vi "Калькулятор.vi"() -> ()   [LabVIEW 2012]
uses:
  Control 1.ctl
panel:
  in  "Backsppace":bool
  in  "CE":bool
  in  "+/-":bool
  in  ",":bool
  in  "1/x":bool
  in  "кв":bool
  in  "к":bool
  in  "MC":bool
  out "Boolean":bool
  in  "MR":bool
  in  "-":bool
  in  "6":bool
  in  "5":bool
  in  "4":bool
  in  "MS":bool
  in  "С":bool
  in  "/":bool
  in  "*":bool
  in  "0":bool
  in  "9":bool
  in  "8":bool
  in  "7":bool
  in  "3":bool
  in  "stop":bool
  in  "=":bool
  in  "2":bool
  in  "+":bool
  out "екран":string
  in  "1":bool
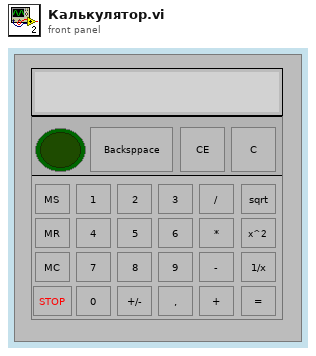
[diagram p1: front panel]
types:
  T1 = typedef "Control 1.ctl" = enum16{"Backspace", "се", "+/-", "т", "1/x", "кв", "к", "mc", "mr", "очистити екран", "ms", "поділити", "помножити", "відняти", "0", "9", "8", "7", "6", "5", "4", "3", "дорівнює", "додати", "2", "1", "евент", "стоп"}
  T2 = cluster{"екран":string, "чистий екран":string, "буфер":string, "Enum":T1, "ms":string, "mr ":string}
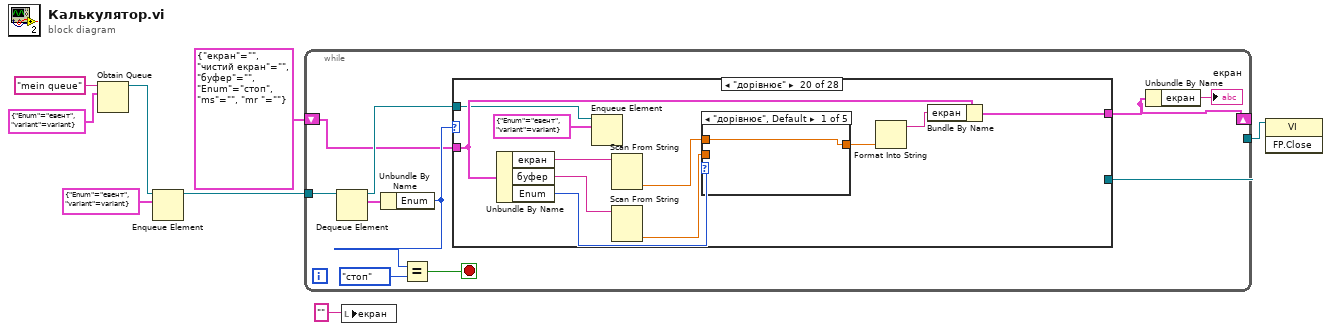
[diagram p0: block diagram]
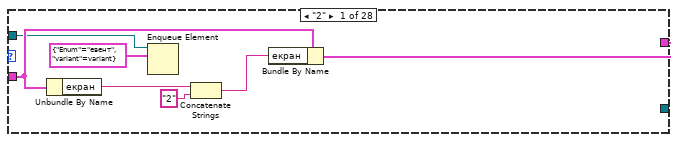
[diagram p2: hidden frame]
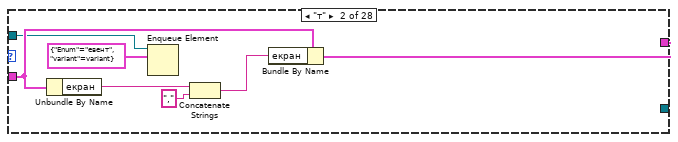
[diagram p3: hidden frame]
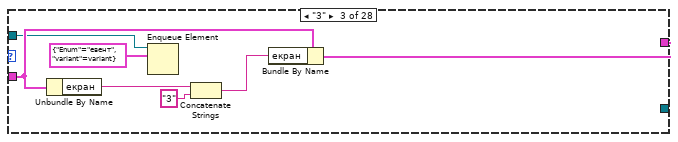
[diagram p4: hidden frame]
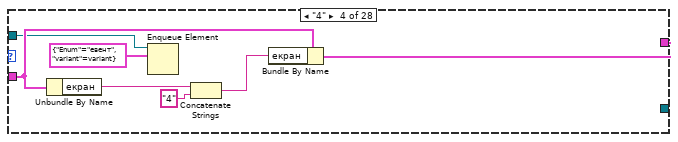
[diagram p5: hidden frame]
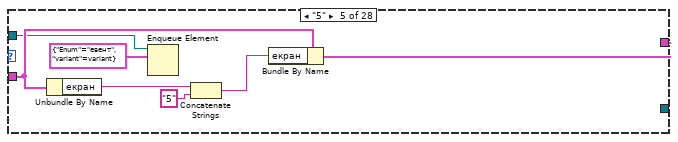
[diagram p6: hidden frame]
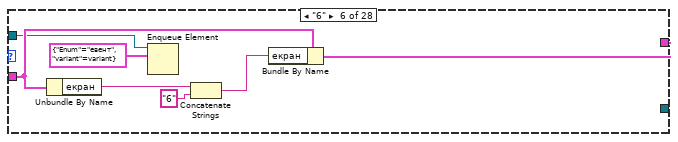
[diagram p7: hidden frame]
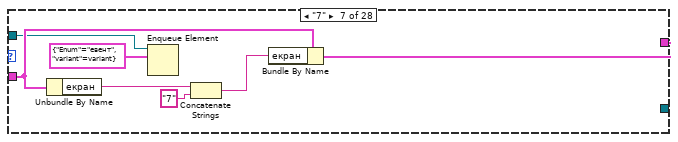
[diagram p8: hidden frame]
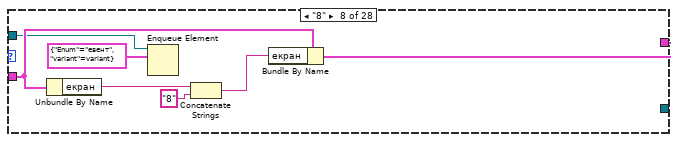
[diagram p9: hidden frame]
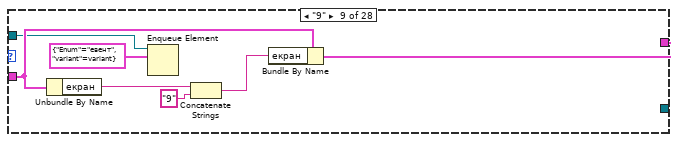
[diagram p10: hidden frame]
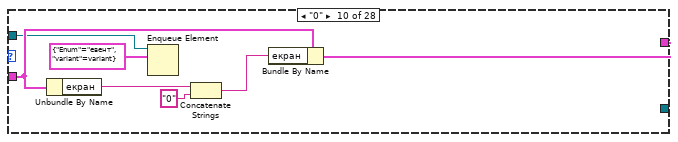
[diagram p11: hidden frame]
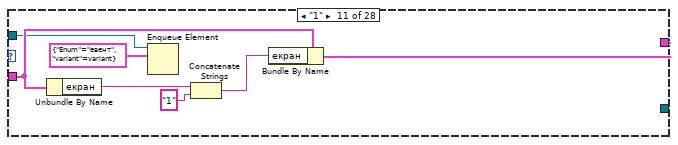
[diagram p12: hidden frame]
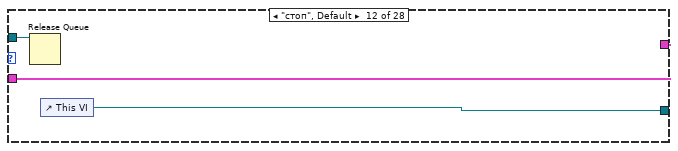
[diagram p13: hidden frame]
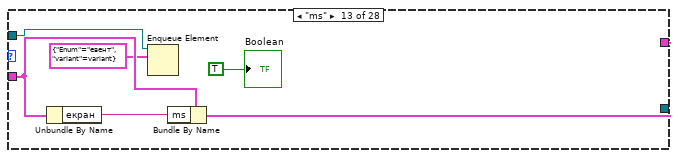
[diagram p14: hidden frame]
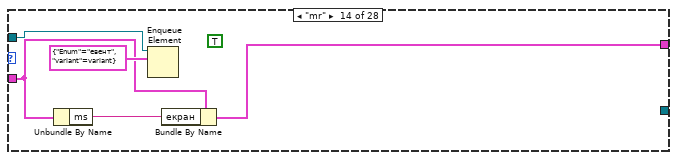
[diagram p15: hidden frame]
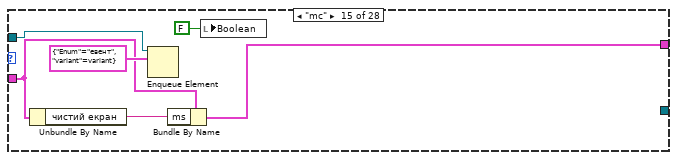
[diagram p16: hidden frame]
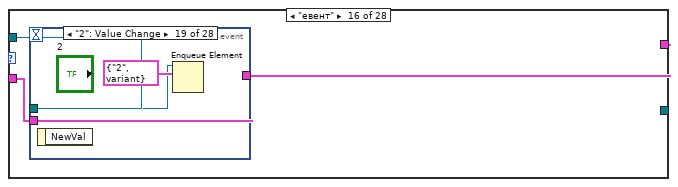
[diagram p17: hidden frame]
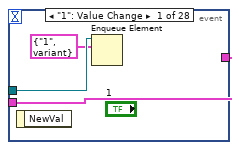
[diagram p18: hidden frame]
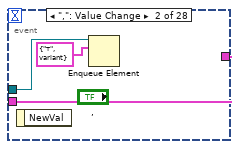
[diagram p19: hidden frame]
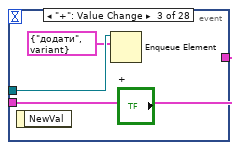
[diagram p20: hidden frame]
diagram:
  n1 = Obtain Queue(name (unnamed)="mein queue", element data type=cluster{"Enum":T1, "variant":variant} {"Enum"=enum."евент", "variant"=variant}) -> (queue out=w7:refnum<queue>)  [unwired: 3 in, 2 out]
  n2 = Enqueue Element(queue=w7, element=cluster{"Enum":T1, "variant":variant} {"Enum"=enum."евент", "variant"=variant}) -> (queue out=w4:refnum<queue>)  [unwired: 2 in, 2 out]
  n3 = while {
    tunnel: w4 -> [w16]
    shift-right: [w11] -> _
    shift-left: T2 {"екран"="", "чистий екран"="", "буфер"="", "Enum"=enum."стоп", "ms"="", "mr "=""} -> [w12]
    tunnel: [w9] -> w2
    stop <- w17 stop-if-true
    n4 = Dequeue Element(queue=w16) -> (queue out=w13:refnum<queue>, element=w15:cluster{"Enum":T1, "variant":variant})  [unwired: 2 in, 2 out]
    n5 = Unbundle By Name(w15) -> ("Enum"=w14:T1)
    n6 = Equal?(x=w14, y=Control_1."стоп" ("Enum")) -> (x = y?=w17:bool)
    n7 = case shown="\"дорівнює\"" w14 {
      tunnel: w13 -> [w20 w27 w34 w41 w48 w55 w62 w69 w76 w83 w90 w97 w100 w109 w115 w118 w237 w238 w250 w253 w282 w284 w297 w309 w317 w324 w331 w338]
      tunnel: w12 -> [w23 w30 w37 w44 w51 w58 w65 w72 w79 w86 w93 w98 w104 w106 w112 w116 w235 w242 w246 w257 w281 w286 w296 w308 w316 w323 w330 w337]
      tunnel: [w22 w29 w36 w43 w50 w57 w64 w71 w78 w85 w91 w98 w103 w105 w111 w117 w234 w240 w244 w256 w276 w285 w294 w306 w314 w318 w325 w332] -> w11
      tunnel: [_ _ _ _ _ _ _ _ _ _ _ w96 _ _ _ _ _ _ _ _ _ _ _ _ _ _ _ _] -> w9
      frame "2" {
        n8 = Unbundle By Name(w23) -> ("екран"=w25:string)
        n9 = Enqueue Element(queue=w20, element=cluster{"Enum":T1, "variant":variant} {"Enum"=enum."евент", "variant"=variant}) -> ()  [unwired: 2 in, 3 out]
        n10 = Concatenate Strings(w25, "2" ("string")) -> (w21:string)
        n11 = Bundle By Name(cluster=w23, "екран"=w21) -> (w22:T2)
      }
      frame "т" {
        n12 = Unbundle By Name(w30) -> ("екран"=w32:string)
        n13 = Enqueue Element(queue=w27, element=cluster{"Enum":T1, "variant":variant} {"Enum"=enum."евент", "variant"=variant}) -> ()  [unwired: 2 in, 3 out]
        n14 = Concatenate Strings(w32, "," ("string")) -> (w28:string)
        n15 = Bundle By Name(cluster=w30, "екран"=w28) -> (w29:T2)
      }
      frame "3" {
        n16 = Unbundle By Name(w37) -> ("екран"=w39:string)
        n17 = Enqueue Element(queue=w34, element=cluster{"Enum":T1, "variant":variant} {"Enum"=enum."евент", "variant"=variant}) -> ()  [unwired: 2 in, 3 out]
        n18 = Concatenate Strings(w39, "3" ("string")) -> (w35:string)
        n19 = Bundle By Name(cluster=w37, "екран"=w35) -> (w36:T2)
      }
      frame "4" {
        n20 = Unbundle By Name(w44) -> ("екран"=w46:string)
        n21 = Enqueue Element(queue=w41, element=cluster{"Enum":T1, "variant":variant} {"Enum"=enum."евент", "variant"=variant}) -> ()  [unwired: 2 in, 3 out]
        n22 = Concatenate Strings(w46, "4" ("string")) -> (w42:string)
        n23 = Bundle By Name(cluster=w44, "екран"=w42) -> (w43:T2)
      }
      frame "5" {
        n24 = Unbundle By Name(w51) -> ("екран"=w53:string)
        n25 = Enqueue Element(queue=w48, element=cluster{"Enum":T1, "variant":variant} {"Enum"=enum."евент", "variant"=variant}) -> ()  [unwired: 2 in, 3 out]
        n26 = Concatenate Strings(w53, "5" ("string")) -> (w49:string)
        n27 = Bundle By Name(cluster=w51, "екран"=w49) -> (w50:T2)
      }
      frame "6" {
        n28 = Unbundle By Name(w58) -> ("екран"=w60:string)
        n29 = Enqueue Element(queue=w55, element=cluster{"Enum":T1, "variant":variant} {"Enum"=enum."евент", "variant"=variant}) -> ()  [unwired: 2 in, 3 out]
        n30 = Concatenate Strings(w60, "6" ("string")) -> (w56:string)
        n31 = Bundle By Name(cluster=w58, "екран"=w56) -> (w57:T2)
      }
      frame "7" {
        n32 = Unbundle By Name(w65) -> ("екран"=w67:string)
        n33 = Enqueue Element(queue=w62, element=cluster{"Enum":T1, "variant":variant} {"Enum"=enum."евент", "variant"=variant}) -> ()  [unwired: 2 in, 3 out]
        n34 = Concatenate Strings(w67, "7" ("string")) -> (w63:string)
        n35 = Bundle By Name(cluster=w65, "екран"=w63) -> (w64:T2)
      }
      frame "8" {
        n36 = Unbundle By Name(w72) -> ("екран"=w74:string)
        n37 = Enqueue Element(queue=w69, element=cluster{"Enum":T1, "variant":variant} {"Enum"=enum."евент", "variant"=variant}) -> ()  [unwired: 2 in, 3 out]
        n38 = Concatenate Strings(w74, "8" ("string")) -> (w70:string)
        n39 = Bundle By Name(cluster=w72, "екран"=w70) -> (w71:T2)
      }
      frame "9" {
        n40 = Unbundle By Name(w79) -> ("екран"=w81:string)
        n41 = Enqueue Element(queue=w76, element=cluster{"Enum":T1, "variant":variant} {"Enum"=enum."евент", "variant"=variant}) -> ()  [unwired: 2 in, 3 out]
        n42 = Concatenate Strings(w81, "9" ("string")) -> (w77:string)
        n43 = Bundle By Name(cluster=w79, "екран"=w77) -> (w78:T2)
      }
      frame "0" {
        n44 = Unbundle By Name(w86) -> ("екран"=w88:string)
        n45 = Enqueue Element(queue=w83, element=cluster{"Enum":T1, "variant":variant} {"Enum"=enum."евент", "variant"=variant}) -> ()  [unwired: 2 in, 3 out]
        n46 = Concatenate Strings(w88, "0" ("string")) -> (w84:string)
        n47 = Bundle By Name(cluster=w86, "екран"=w84) -> (w85:T2)
      }
      frame "1" {
        n48 = Unbundle By Name(w93) -> ("екран"=w95:string)
        n49 = Enqueue Element(queue=w90, element=cluster{"Enum":T1, "variant":variant} {"Enum"=enum."евент", "variant"=variant}) -> ()  [unwired: 2 in, 3 out]
        n50 = Concatenate Strings(w95, "1" ("string")) -> (w92:string)
        n51 = Bundle By Name(cluster=w93, "екран"=w92) -> (w91:T2)
      }
      frame "стоп", Default {
        n52 = Release Queue(queue=w97) -> ()  [unwired: 2 in, 3 out]
        n53 = control-ref of="This VI"() -> (w96:refnum<vi>)
      }
      frame "ms" {
        n54 = Unbundle By Name(w104) -> ("екран"=w101:string)
        n55 = Enqueue Element(queue=w100, element=cluster{"Enum":T1, "variant":variant} {"Enum"=enum."евент", "variant"=variant}) -> ()  [unwired: 2 in, 3 out]
        n56 = Bundle By Name(cluster=w104, "ms"=w101) -> (w103:T2)
        "Boolean" <- TRUE
      }
      frame "mr" {
        (unwired) TRUE
        n57 = Unbundle By Name(w106) -> ("ms"=w107:string)
        n58 = Enqueue Element(queue=w109, element=cluster{"Enum":T1, "variant":variant} {"Enum"=enum."евент", "variant"=variant}) -> ()  [unwired: 2 in, 3 out]
        n59 = Bundle By Name(cluster=w106, "екран"=w107) -> (w105:T2)
      }
      frame "mc" {
        n60 = Unbundle By Name(w112) -> ("чистий екран"=w113:string)
        n61 = Enqueue Element(queue=w115, element=cluster{"Enum":T1, "variant":variant} {"Enum"=enum."евент", "variant"=variant}) -> ()  [unwired: 2 in, 3 out]
        n62 = Bundle By Name(cluster=w112, "ms"=w113) -> (w111:T2)
        n63 = local write "Boolean"(FALSE) -> ()
      }
      frame "евент" {
        n64 = event shown="[18] \"2\": Value Change" {
          selector: _ -> [_ _ _ _ _ _ _ _ _ _ _ _ _ _ _ _ _ _ _ _ _ _ _ _ _ _ _ _]
          dyn-events: _ -> [_ _ _ _ _ _ _ _ _ _ _ _ _ _ _ _ _ _ _ _ _ _ _ _ _ _ _ _]
          timeout: _ -> [_ _ _ _ _ _ _ _ _ _ _ _ _ _ _ _ _ _ _ _ _ _ _ _ _ _ _ _]
          tunnel: w118 -> [w121 w124 w126 w129 w132 w135 w138 w141 w144 w147 w151 w153 w156 w159 w162 w165 w168 w171 w201 w204 w207 w210 w213 w216 w219 w222 w225 w228]
          tunnel: [w119 w122 w127 w130 w133 w136 w139 w142 w145 w148 w149 w152 w155 w158 w161 w166 w167 w170 w203 w206 w209 w212 w215 w218 w221 w224 w227 w230] -> w117
          tunnel: w116 -> [w119 w122 w127 w130 w133 w136 w139 w142 w145 w148 w149 w152 w155 w158 w161 w166 w167 w170 w203 w206 w209 w212 w215 w218 w221 w224 w227 w230]
          event "1": Value Change {
            n65 = event-data() -> ()  [unwired: 1 in, 1 out]
            n66 = Enqueue Element(queue=w121, element=cluster{"Enum":T1, "variant":variant} {"Enum"=enum."1", "variant"=variant}) -> ()  [unwired: 2 in, 3 out]
          }
          event ",": Value Change {
            n67 = event-data() -> ()  [unwired: 1 in, 1 out]
            n68 = Enqueue Element(queue=w124, element=cluster{"Enum":T1, "variant":variant} {"Enum"=enum."т", "variant"=variant}) -> ()  [unwired: 2 in, 3 out]
          }
          event "+": Value Change {
            n69 = event-data() -> ()  [unwired: 1 in, 1 out]
            n70 = Enqueue Element(queue=w126, element=cluster{"Enum":T1, "variant":variant} {"Enum"=enum."додати", "variant"=variant}) -> ()  [unwired: 2 in, 3 out]
          }
          event "к": Value Change {
            n71 = event-data() -> ()  [unwired: 1 in, 1 out]
            n72 = Enqueue Element(queue=w129, element=cluster{"Enum":T1, "variant":variant} {"Enum"=enum."к", "variant"=variant}) -> ()  [unwired: 2 in, 3 out]
          }
          event "кв": Value Change {
            n73 = event-data() -> ()  [unwired: 1 in, 1 out]
            n74 = Enqueue Element(queue=w132, element=cluster{"Enum":T1, "variant":variant} {"Enum"=enum."кв", "variant"=variant}) -> ()  [unwired: 2 in, 3 out]
          }
          event "1/x": Value Change {
            n75 = event-data() -> ()  [unwired: 1 in, 1 out]
            n76 = Enqueue Element(queue=w135, element=cluster{"Enum":T1, "variant":variant} {"Enum"=enum."1/x", "variant"=variant}) -> ()  [unwired: 2 in, 3 out]
          }
          event "С": Value Change {
            n77 = event-data() -> ()  [unwired: 1 in, 1 out]
            n78 = Enqueue Element(queue=w138, element=cluster{"Enum":T1, "variant":variant} {"Enum"=enum."очистити екран", "variant"=variant}) -> ()  [unwired: 2 in, 3 out]
          }
          event "-": Value Change {
            n79 = event-data() -> ()  [unwired: 1 in, 1 out]
            n80 = Enqueue Element(queue=w141, element=cluster{"Enum":T1, "variant":variant} {"Enum"=enum."відняти", "variant"=variant}) -> ()  [unwired: 2 in, 3 out]
          }
          event "*": Value Change {
            n81 = event-data() -> ()  [unwired: 1 in, 1 out]
            n82 = Enqueue Element(queue=w144, element=cluster{"Enum":T1, "variant":variant} {"Enum"=enum."помножити", "variant"=variant}) -> ()  [unwired: 2 in, 3 out]
          }
          event "/": Value Change {
            n83 = event-data() -> ()  [unwired: 1 in, 1 out]
            n84 = Enqueue Element(queue=w147, element=cluster{"Enum":T1, "variant":variant} {"Enum"=enum."поділити", "variant"=variant}) -> ()  [unwired: 2 in, 3 out]
          }
          event "CE": Value Change {
            n85 = event-data() -> ()  [unwired: 1 in, 1 out]
            n86 = Enqueue Element(queue=w151, element=cluster{"Enum":T1, "variant":variant} {"Enum"=enum."се", "variant"=variant}) -> ()  [unwired: 2 in, 3 out]
          }
          event "MS": Value Change {
            n87 = event-data() -> ()  [unwired: 1 in, 1 out]
            n88 = Enqueue Element(queue=w153, element=cluster{"Enum":T1, "variant":variant} {"Enum"=enum."ms", "variant"=variant}) -> ()  [unwired: 2 in, 3 out]
          }
          event "MC": Value Change {
            n89 = event-data() -> ()  [unwired: 1 in, 1 out]
            n90 = Enqueue Element(queue=w156, element=cluster{"Enum":T1, "variant":variant} {"Enum"=enum."mc", "variant"=variant}) -> ()  [unwired: 2 in, 3 out]
          }
          event "Backsppace": Value Change {
            n91 = event-data() -> ()  [unwired: 1 in, 1 out]
            n92 = Enqueue Element(queue=w159, element=cluster{"Enum":T1, "variant":variant} {"Enum"=enum."Backspace", "variant"=variant}) -> ()  [unwired: 2 in, 3 out]
          }
          event "MR": Value Change {
            n93 = event-data() -> ()  [unwired: 1 in, 1 out]
            n94 = Enqueue Element(queue=w162, element=cluster{"Enum":T1, "variant":variant} {"Enum"=enum."mr", "variant"=variant}) -> ()  [unwired: 2 in, 3 out]
          }
          event "=": Value Change {
            n95 = event-data() -> ()  [unwired: 1 in, 1 out]
            n96 = Enqueue Element(queue=w165, element=cluster{"Enum":T1, "variant":variant} {"Enum"=enum."дорівнює", "variant"=variant}) -> ()  [unwired: 2 in, 3 out]
          }
          event "+/-": Value Change {
            n97 = event-data() -> ()  [unwired: 1 in, 1 out]
            n98 = Enqueue Element(queue=w168, element=cluster{"Enum":T1, "variant":variant} {"Enum"=enum."+/-", "variant"=variant}) -> ()  [unwired: 2 in, 3 out]
          }
          event Menu Selection (User) {
            n99 = event-data() -> ("ItemTag"=w172:string)  [unwired: 1 in]
            n100 = case shown="\"додати до пам'яті\"" w172 {
              tunnel: w171 -> [_ w174 w176 w178 w180 w182 w184 w186 w188 w190 w192 w194 w196 w198 w200]
              frame "False", Default {
              }
              frame "стоп" {
                n101 = Enqueue Element(queue=w174, element=cluster{"Enum":T1, "variant":variant} {"Enum"=enum."стоп", "variant"=variant}) -> ()  [unwired: 2 in, 3 out]
              }
              frame "додати" {
                n102 = Enqueue Element(queue=w176, element=cluster{"Enum":T1, "variant":variant} {"Enum"=enum."додати", "variant"=variant}) -> ()  [unwired: 2 in, 3 out]
              }
              frame "відняти" {
                n103 = Enqueue Element(queue=w178, element=cluster{"Enum":T1, "variant":variant} {"Enum"=enum."відняти", "variant"=variant}) -> ()  [unwired: 2 in, 3 out]
              }
              frame "поділити" {
                n104 = Enqueue Element(queue=w180, element=cluster{"Enum":T1, "variant":variant} {"Enum"=enum."поділити", "variant"=variant}) -> ()  [unwired: 2 in, 3 out]
              }
              frame "помножити" {
                n105 = Enqueue Element(queue=w182, element=cluster{"Enum":T1, "variant":variant} {"Enum"=enum."помножити", "variant"=variant}) -> ()  [unwired: 2 in, 3 out]
              }
              frame "корінь квадратний" {
                n106 = Enqueue Element(queue=w184, element=cluster{"Enum":T1, "variant":variant} {"Enum"=enum."к", "variant"=variant}) -> ()  [unwired: 2 in, 3 out]
              }
              frame "квадрат" {
                n107 = Enqueue Element(queue=w186, element=cluster{"Enum":T1, "variant":variant} {"Enum"=enum."кв", "variant"=variant}) -> ()  [unwired: 2 in, 3 out]
              }
              frame "1/х" {
                n108 = Enqueue Element(queue=w188, element=cluster{"Enum":T1, "variant":variant} {"Enum"=enum."1/x", "variant"=variant}) -> ()  [unwired: 2 in, 3 out]
              }
              frame "+/-" {
                n109 = Enqueue Element(queue=w190, element=cluster{"Enum":T1, "variant":variant} {"Enum"=enum."+/-", "variant"=variant}) -> ()  [unwired: 2 in, 3 out]
              }
              frame "додати до пам'яті" {
                n110 = Enqueue Element(queue=w192, element=cluster{"Enum":T1, "variant":variant} {"Enum"=enum."ms", "variant"=variant}) -> ()  [unwired: 2 in, 3 out]
              }
              frame "вивести на екран" {
                n111 = Enqueue Element(queue=w194, element=cluster{"Enum":T1, "variant":variant} {"Enum"=enum."mr", "variant"=variant}) -> ()  [unwired: 2 in, 3 out]
              }
              frame "очистити пам'ять" {
                n112 = Enqueue Element(queue=w196, element=cluster{"Enum":T1, "variant":variant} {"Enum"=enum."mc", "variant"=variant}) -> ()  [unwired: 2 in, 3 out]
              }
              frame "екран (с)" {
                n113 = Enqueue Element(queue=w198, element=cluster{"Enum":T1, "variant":variant} {"Enum"=enum."очистити екран", "variant"=variant}) -> ()  [unwired: 2 in, 3 out]
              }
              frame "буфер (CE)" {
                n114 = Enqueue Element(queue=w200, element=cluster{"Enum":T1, "variant":variant} {"Enum"=enum."се", "variant"=variant}) -> ()  [unwired: 2 in, 3 out]
              }
            }
          }
          event "2": Value Change {
            n115 = event-data() -> ()  [unwired: 1 in, 1 out]
            n116 = Enqueue Element(queue=w201, element=cluster{"Enum":T1, "variant":variant} {"Enum"=enum."2", "variant"=variant}) -> ()  [unwired: 2 in, 3 out]
          }
          event "3": Value Change {
            n117 = event-data() -> ()  [unwired: 1 in, 1 out]
            n118 = Enqueue Element(queue=w204, element=cluster{"Enum":T1, "variant":variant} {"Enum"=enum."3", "variant"=variant}) -> ()  [unwired: 2 in, 3 out]
          }
          event "4": Value Change {
            n119 = event-data() -> ()  [unwired: 1 in, 1 out]
            n120 = Enqueue Element(queue=w207, element=cluster{"Enum":T1, "variant":variant} {"Enum"=enum."4", "variant"=variant}) -> ()  [unwired: 2 in, 3 out]
          }
          event "5": Value Change {
            n121 = event-data() -> ()  [unwired: 1 in, 1 out]
            n122 = Enqueue Element(queue=w210, element=cluster{"Enum":T1, "variant":variant} {"Enum"=enum."5", "variant"=variant}) -> ()  [unwired: 2 in, 3 out]
          }
          event "6": Value Change {
            n123 = event-data() -> ()  [unwired: 1 in, 1 out]
            n124 = Enqueue Element(queue=w213, element=cluster{"Enum":T1, "variant":variant} {"Enum"=enum."6", "variant"=variant}) -> ()  [unwired: 2 in, 3 out]
          }
          event "7": Value Change {
            n125 = event-data() -> ()  [unwired: 1 in, 1 out]
            n126 = Enqueue Element(queue=w216, element=cluster{"Enum":T1, "variant":variant} {"Enum"=enum."7", "variant"=variant}) -> ()  [unwired: 2 in, 3 out]
          }
          event "8": Value Change {
            n127 = event-data() -> ()  [unwired: 1 in, 1 out]
            n128 = Enqueue Element(queue=w219, element=cluster{"Enum":T1, "variant":variant} {"Enum"=enum."8", "variant"=variant}) -> ()  [unwired: 2 in, 3 out]
          }
          event "9": Value Change {
            n129 = event-data() -> ()  [unwired: 1 in, 1 out]
            n130 = Enqueue Element(queue=w222, element=cluster{"Enum":T1, "variant":variant} {"Enum"=enum."9", "variant"=variant}) -> ()  [unwired: 2 in, 3 out]
          }
          event "0": Value Change {
            n131 = event-data() -> ()  [unwired: 1 in, 1 out]
            n132 = Enqueue Element(queue=w225, element=cluster{"Enum":T1, "variant":variant} {"Enum"=enum."0", "variant"=variant}) -> ()  [unwired: 2 in, 3 out]
          }
          event "stop": Value Change {
            n133 = event-data() -> ()  [unwired: 1 in, 1 out]
            n134 = Enqueue Element(queue=w228, element=cluster{"Enum":T1, "variant":variant} {"Enum"=enum."стоп", "variant"=variant}) -> ()  [unwired: 2 in, 3 out]
          }
        }
      }
      frame "+/-" {
        n135 = Unbundle By Name(w235) -> ("екран"=w233:string)
        n136 = Enqueue Element(queue=w237, element=cluster{"Enum":T1, "variant":variant} {"Enum"=enum."евент", "variant"=variant}) -> ()  [unwired: 2 in, 3 out]
        n137 = Concatenate Strings("-" ("string"), w233) -> (w231:string)
        n138 = Bundle By Name(cluster=w235, "екран"=w231) -> (w234:T2)
      }
      frame "очистити екран" {
        n139 = Unbundle By Name(w242) -> ("чистий екран"=w241:string)
        n140 = Enqueue Element(queue=w238, element=cluster{"Enum":T1, "variant":variant} {"Enum"=enum."евент", "variant"=variant}) -> ()  [unwired: 2 in, 3 out]
        n141 = Bundle By Name(cluster=w242, "екран"=w241, "буфер"=w241) -> (w240:T2)
      }
      frame "Backspace" {
        n142 = Unbundle By Name(w246) -> ("екран"=w243:string)
        n143 = Enqueue Element(queue=w250, element=cluster{"Enum":T1, "variant":variant} {"Enum"=enum."евент", "variant"=variant}) -> ()  [unwired: 2 in, 3 out]
        n144 = String Length(string=w243) -> (length=w249:i32)
        n145 = Subtract(x=w249, y=1) -> (x-y=w247:i32)
        n146 = String Subset(string=w243, length (rest)=w247) -> (substring=w245:string)  [unwired: 1 in]
        n147 = Bundle By Name(cluster=w246, "екран"=w245) -> (w244:T2)
      }
      frame "дорівнює" {
        n148 = Unbundle By Name(w257) -> ("екран"=w262:string, "буфер"=w261:string, "Enum"=w260:T1)
        n149 = Enqueue Element(queue=w253, element=cluster{"Enum":T1, "variant":variant} {"Enum"=enum."евент", "variant"=variant}) -> ()  [unwired: 2 in, 3 out]
        n150 = Scan From String(input string=w262) -> (output 1=w258:dbl)  [unwired: 4 in, 3 out]
        n151 = Scan From String(input string=w261) -> (output 1=w259:dbl)  [unwired: 4 in, 3 out]
        n152 = case shown="\"дорівнює\", Default" w260 {
          tunnel: w259 -> [_ w266 w267 w270 w273]
          tunnel: w258 -> [w263 w265 w268 w271 w274]
          tunnel: [w263 w264 w269 w272 w275] -> w255
          frame "дорівнює", Default {
          }
          frame "додати" {
            n153 = Add(x=w265, y=w266) -> (x+y=w264:dbl)
          }
          frame "відняти" {
            n154 = Subtract(x=w267, y=w268) -> (x-y=w269:dbl)
          }
          frame "поділити" {
            n155 = Divide(x=w270, y=w271) -> (x/y=w272:dbl)
          }
          frame "помножити" {
            n156 = Multiply(x=w274, y=w273) -> (x*y=w275:dbl)
          }
        }
        n157 = Format Into String(w255) -> (resulting string=w254:string)  [unwired: 3 in, 1 out]
        n158 = Bundle By Name(cluster=w257, "екран"=w254) -> (w256:T2)
      }
      frame "додати" {
        n159 = Unbundle By Name(w281) -> ("екран"=w280:string, "чистий екран"=w279:string)
        n160 = Enqueue Element(queue=w282, element=cluster{"Enum":T1, "variant":variant} {"Enum"=enum."евент", "variant"=variant}) -> ()  [unwired: 2 in, 3 out]
        n161 = Bundle By Name(cluster=w281, "буфер"=w280, "екран"=w279, "Enum"=Control_1."додати") -> (w276:T2)
      }
      frame "се" {
        n162 = Unbundle By Name(w286) -> ("чистий екран"=w287:string)
        n163 = Enqueue Element(queue=w284, element=cluster{"Enum":T1, "variant":variant} {"Enum"=enum."евент", "variant"=variant}) -> ()  [unwired: 2 in, 3 out]
        n164 = Bundle By Name(cluster=w286, "екран"=w287) -> (w285:T2)
      }
      frame "к" {
        n165 = Unbundle By Name(w296) -> ("екран"=w293:string)
        n166 = Enqueue Element(queue=w297, element=cluster{"Enum":T1, "variant":variant} {"Enum"=enum."евент", "variant"=variant}) -> ()  [unwired: 2 in, 3 out]
        n167 = Scan From String(input string=w293) -> (output 1=w289:dbl)  [unwired: 4 in, 3 out]
        n168 = Greater?(x=w289, y=0.0) -> (0:w290:bool)
        n169 = case shown="False" w290 {
          tunnel: w289 -> [_ w301]
          tunnel: [0.0 w300] -> w288
          frame False {
            n170 = One Button Dialog(message="корінь з від'ємного числа не існує") -> ()  [unwired: 1 in, 1 out]
          }
          frame True {
            n171 = Square Root(x=w301) -> (sqrt(x)=w300:dbl)
          }
        }
        n172 = Format Into String(w288) -> (resulting string=w292:string)  [unwired: 3 in, 1 out]
        n173 = Bundle By Name(cluster=w296, "екран"=w292) -> (w294:T2)
      }
      frame "1/x" {
        n174 = Unbundle By Name(w308) -> ("екран"=w305:string)
        n175 = Enqueue Element(queue=w309, element=cluster{"Enum":T1, "variant":variant} {"Enum"=enum."евент", "variant"=variant}) -> ()  [unwired: 2 in, 3 out]
        n176 = Scan From String(input string=w305) -> (output 1=w303:dbl)  [unwired: 4 in, 3 out]
        n177 = Reciprocal(x=w303) -> (1/x=w302:dbl)
        n178 = Format Into String(w302) -> (resulting string=w304:string)  [unwired: 3 in, 1 out]
        n179 = Bundle By Name(cluster=w308, "екран"=w304) -> (w306:T2)
      }
      frame "кв" {
        n180 = Unbundle By Name(w316) -> ("екран"=w313:string)
        n181 = Enqueue Element(queue=w317, element=cluster{"Enum":T1, "variant":variant} {"Enum"=enum."евент", "variant"=variant}) -> ()  [unwired: 2 in, 3 out]
        n182 = Scan From String(input string=w313) -> (output 1=w311:dbl)  [unwired: 4 in, 3 out]
        n183 = Square(x=w311) -> (x^2=w310:dbl)
        n184 = Format Into String(w310) -> (resulting string=w312:string)  [unwired: 3 in, 1 out]
        n185 = Bundle By Name(cluster=w316, "екран"=w312) -> (w314:T2)
      }
      frame "поділити" {
        n186 = Unbundle By Name(w323) -> ("екран"=w322:string, "чистий екран"=w321:string)
        n187 = Enqueue Element(queue=w324, element=cluster{"Enum":T1, "variant":variant} {"Enum"=enum."евент", "variant"=variant}) -> ()  [unwired: 2 in, 3 out]
        n188 = Bundle By Name(cluster=w323, "буфер"=w322, "екран"=w321, "Enum"=Control_1."поділити") -> (w318:T2)
      }
      frame "помножити" {
        n189 = Unbundle By Name(w330) -> ("екран"=w329:string, "чистий екран"=w328:string)
        n190 = Enqueue Element(queue=w331, element=cluster{"Enum":T1, "variant":variant} {"Enum"=enum."евент", "variant"=variant}) -> ()  [unwired: 2 in, 3 out]
        n191 = Bundle By Name(cluster=w330, "буфер"=w329, "екран"=w328, "Enum"=Control_1."помножити") -> (w325:T2)
      }
      frame "відняти" {
        n192 = Unbundle By Name(w337) -> ("екран"=w336:string, "чистий екран"=w335:string)
        n193 = Enqueue Element(queue=w338, element=cluster{"Enum":T1, "variant":variant} {"Enum"=enum."евент", "variant"=variant}) -> ()  [unwired: 2 in, 3 out]
        n194 = Bundle By Name(cluster=w337, "буфер"=w336, "екран"=w335, "Enum"=Control_1."відняти") -> (w332:T2)
      }
    }
    n195 = Unbundle By Name(w11) -> ("екран"=→"екран":string)
  }
  n196 = local write "екран"("" ("екран")) -> ()
  n197 = invoke class="VI" method="FP.Close"(reference=w2) -> ()  [unwired: 2 in, 3 out]
